vi "Aquire Data.vi"(8 "error in (no error)":errorcluster, 9 "Data Save Location":path, 10 "Aqusition Time (s)":dbl, 11 "Aquire Data in":refnum<class "Aquire Data.lvclass">) -> (0 "error out":errorcluster, 3 "Aquire Data out":refnum<class "Aquire Data.lvclass">)   [LabVIEW 2022 SP3, in "Aquire Data.lvclass"]
uses:
  Aquire Data.lvclass
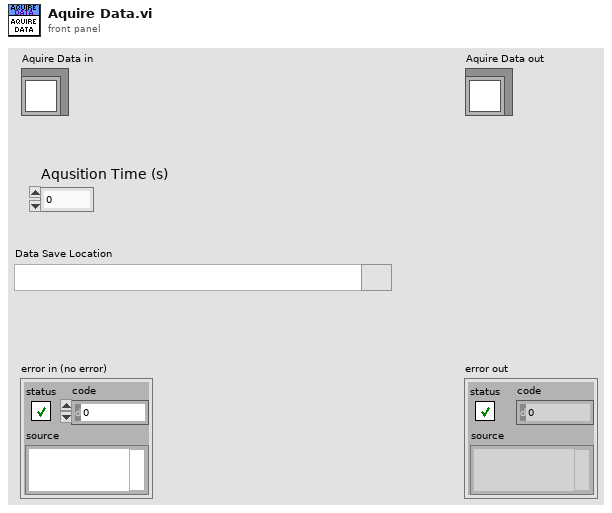
[diagram p1: front panel]
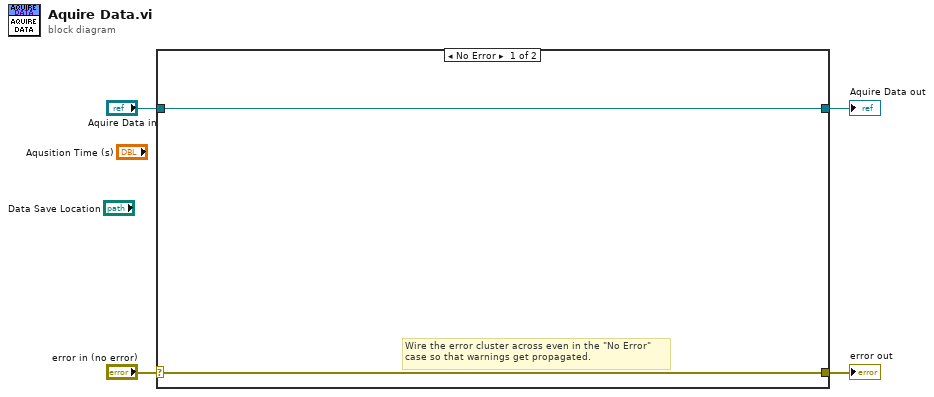
[diagram p0: block diagram]
diagram:
  n1 = case shown="No Error" "error in (no error)" {
    selector: "error in (no error)" -> [w5 w8]
    tunnel: [w5 w8] -> w3
    tunnel: [w6 w7] -> w1
    tunnel: "Aquire Data in" -> [w6 w7]
    frame No Error {
      # "Wire the error cluster across even in the \"No Error\"\ncase so that warnings get propagated."
    }
    frame Error {
    }
  }
  "error out" <- w3
  "Aquire Data out" <- w1
